vi "onCreateListener.vi"(6 "timeout (ms)":i32=100, 8 "error in (no error)":errorcluster, 10 "Configuration":refnum<class "Connection.lvclass">) -> (0 "error out":errorcluster, 3 "Listener":refnum<class "Connection.lvclass">)   [LabVIEW 2013, in "MQTT_Connection.lvlib" / "Connection.lvclass"]
uses:
  Connection.lvclass
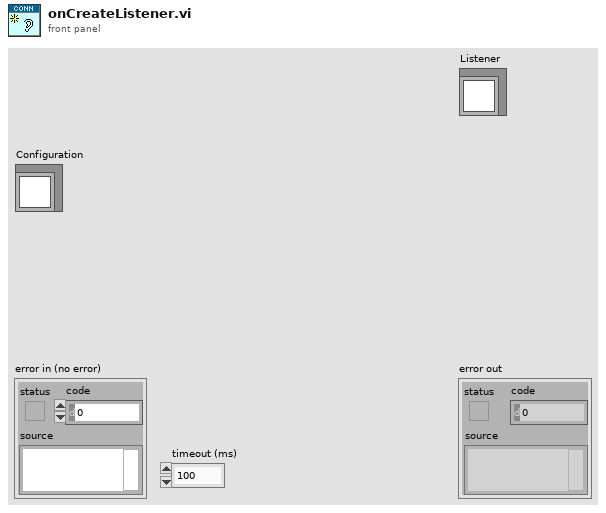
[diagram p1: front panel]
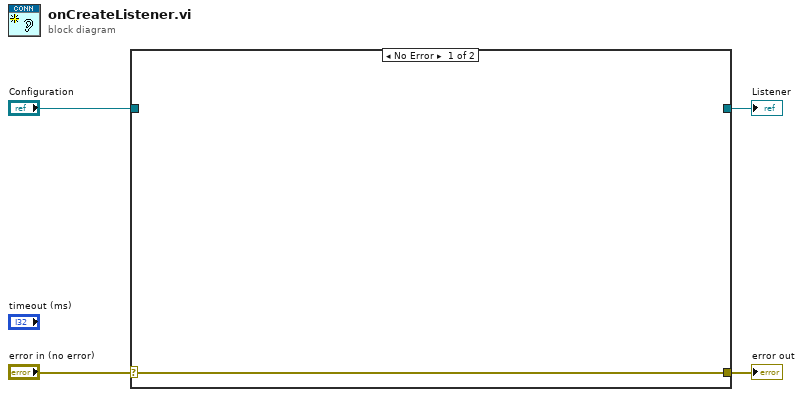
[diagram p0: block diagram]
diagram:
  n1 = case shown="No Error" "error in (no error)" {
    selector: "error in (no error)" -> [w5 w7]
    tunnel: [w5 w7] -> w3
    tunnel: [_ w6] -> w1
    tunnel: "Configuration" -> [_ w6]
    frame No Error {
    }
    frame Error {
    }
  }
  "error out" <- w3
  "Listener" <- w1
